vi "_word.table.FillCells.vi"(7 "word.application":refnum<k7>, 8 "error in (no error)":errorcluster, 9 "start cell":cluster{"x+1":i32, "x+1":i32}, 10 "table row contents":string[][](array[string]), 11 "table in":refnum<k7>) -> (0 "error out":errorcluster, 3 "table out":refnum<k7>)   [LabVIEW 2018, in "WordReportGeneration.lvlib"]
uses:
  WordReportGeneration.lvlib
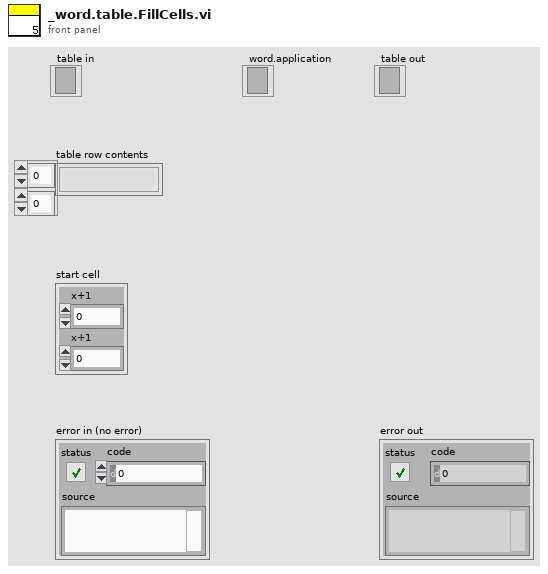
[diagram p1: front panel]
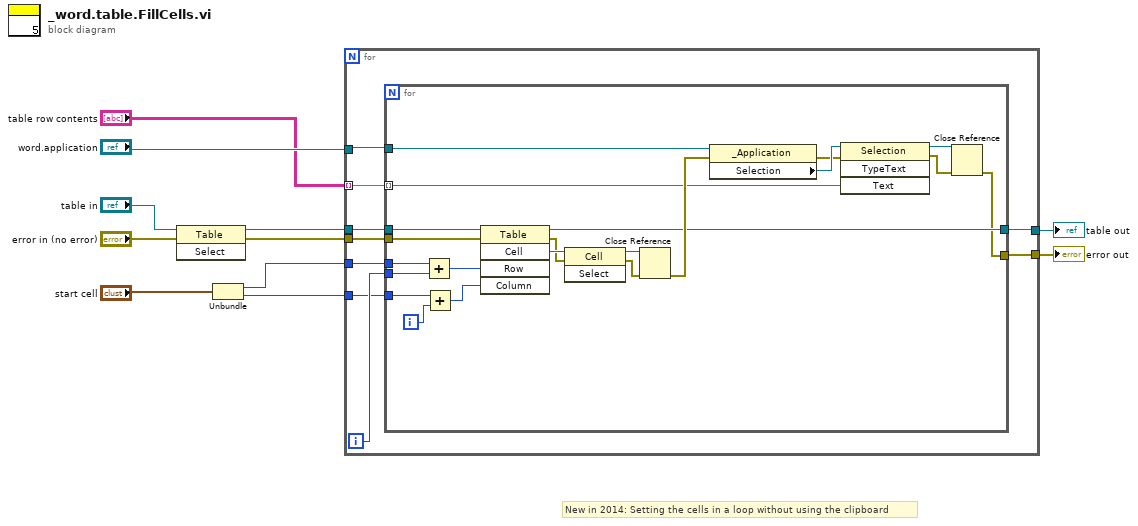
[diagram p0: block diagram]
diagram:
  # "New in 2014: Setting the cells in a loop without using the clipboard"
  n1 = invoke on="Invoke Node" class="Table" method="Select"(reference="table in", error in="error in (no error)") -> (reference out=w9:refnum<k7>, error out=w10:errorcluster)  [unwired: 1 in, 1 out]
  n2 = Unbundle("start cell") -> ("x+1"=w2:i32, "x+1"=w1:i32)
  n3 = for {
    tunnel: "table row contents" -> [w20] mode=indexing
    tunnel: [w19] -> w7
    tunnel: [w18] -> w8
    tunnel: w10 -> [w16]
    tunnel: "word.application" -> [w15]
    tunnel: w9 -> [w14]
    tunnel: w2 -> [w13]
    tunnel: w1 -> [w12]
    i -> [w17]
    n4 = for {
      tunnel: w20 -> [w32] mode=indexing
      tunnel: [w36] -> w19
      tunnel: [w29] -> w18
      tunnel: w17 -> [w26]
      tunnel: w16 -> [w35]
      tunnel: w15 -> [w34]
      tunnel: w14 -> [w33]
      tunnel: w13 -> [w24]
      tunnel: w12 -> [w23]
      i -> [w25]
      n5 = Add(x=w24, y=w26) -> (x+y=w22:i32)
      n6 = Add(x=w23, y=w25) -> (x+y=w21:i32)
      n7 = invoke class="Table" method="Cell"(reference=w33, error in=w35, "Row"=w22, "Column"=w21) -> (reference out=w36:refnum<k7>, error out=w40:errorcluster, "Cell"=w41:refnum<k7>)  [unwired: 1 in, 2 out]
      n8 = invoke class="Cell" method="Select"(reference=w41, error in=w40) -> (reference out=w37:refnum<k7>, error out=w39:errorcluster)  [unwired: 1 in, 1 out]
      n9 = Close Reference(reference=w37, error in (no error)=w39) -> (error out=w38:errorcluster)
      n10 = property class="_Application"(reference=w34, error in=w38) -> (error out=w27:errorcluster, "Selection"=w28:refnum<k7>)  [unwired: 1 out]
      n11 = invoke class="Selection" method="TypeText"(reference=w28, error in=w27, "Text"=w32) -> (reference out=w30:refnum<k7>, error out=w31:errorcluster)  [unwired: 1 in, 2 out]
      n12 = Close Reference(reference=w30, error in (no error)=w31) -> (error out=w29:errorcluster)
    }
  }
  "error out" <- w8
  "table out" <- w7
